vi "AMC Dispatch Start.vi"(8 "error in (no error)":errorcluster) -> (0 "error out":errorcluster)   [LabVIEW 2015]
doc: "This VI is used for compatibility with previous versions of the AMC library. Use the AMC VIs located in the <b>Data Communication >> Asynchronous Message Communication</b> palette."
uses:
  <vilib>/NI/AMC/AMC.lvlib
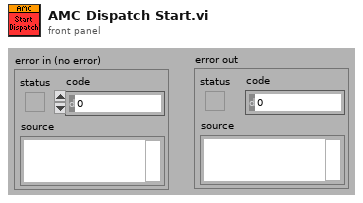
[diagram p1: front panel]
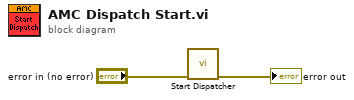
[diagram p0: block diagram]
diagram:
  n1 = call <vilib>:"Start Dispatcher.vi"("error in"="error in (no error)") -> ("error out"=→"error out":errorcluster)  [unwired: 12 in, 2 out]
